vi "update_switch_counter.vi"(0 "PrepLineObject.lvclass":refnum<class "PrepLineObject.lvclass">, 3 "error in (no error)":errorcluster) -> (7 "PrepLineObject out":refnum<class "PrepLineObject.lvclass">, 10 "error out":errorcluster)   [LabVIEW 2018]
doc: "if the switch is turned to true/activated (valve open) the counter in the PrepLineObject is increased by 1. The switch preference file is also being updated"
uses:
  Classes/PrepLineObject/PrepLineObject.lvclass
  <vilib>/Utility/config.llb/Write Key (U32).vi
  <vilib>/Utility/config.llb/NI_LVConfig.lvlib
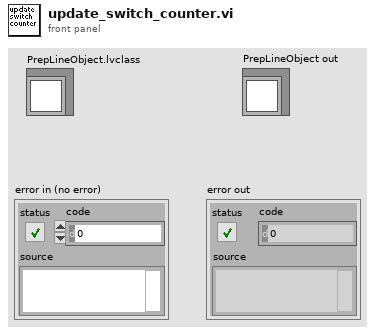
[diagram p1: front panel]
types:
  T1 = typedef "NI_LVConfig.lvlib/Config Data RefNum.ctl" = refnum<k1>
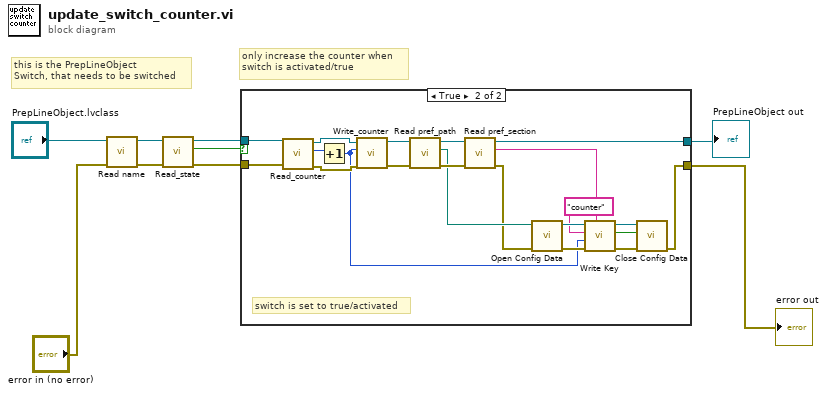
[diagram p0: block diagram]
diagram:
  # "only increase the counter when\nswitch is activated/true"
  # "this is the PrepLineObject\nSwitch, that needs to be switched"
  n1 = call-dynamic "Read name.vi"("error in (no error)"="error in (no error)", "PrepLineObject in"="PrepLineObject.lvclass") -> ("error out"=w7:errorcluster, "PrepLineObject out"=w8:refnum<class "PrepLineObject.lvclass">)  [unwired: 7 in, 1 out]
  n2 = call-dynamic "Read_state.vi"("error in (no error)"=w7, "PrepLineObject in"=w8) -> ("error out"=w5:errorcluster, "state"=w4:bool, "PrepLineObject out"=w6:refnum<class "PrepLineObject.lvclass">)  [unwired: 7 in]
  n3 = case shown="True" w4 {
    tunnel: w6 -> [w11 w29]
    tunnel: w5 -> [w10 w28]
    tunnel: [w11 w23] -> w2
    tunnel: [w10 w12] -> w1
    frame False {
      # "switch is set to false/inactive"
    }
    frame True {
      # "switch is set to true/activated"
      n4 = call-dynamic "Read_counter.vi"("error in (no error)"=w28, "PrepLineObject in"=w29) -> ("error out"=w30:errorcluster, "counter"=w32:u32, "PrepLineObject out"=w31:refnum<class "PrepLineObject.lvclass">)  [unwired: 7 in]
      n5 = Increment(x=w32) -> (x+1=w16:u32)
      n6 = call-dynamic "Write_counter.vi"("error in (no error)"=w30, "counter"=w16, "PrepLineObject in"=w31) -> ("error out"=w26:errorcluster, "PrepLineObject out"=w27:refnum<class "PrepLineObject.lvclass">)  [unwired: 7 in]
      n7 = call-dynamic "Read pref_path.vi"("error in (no error)"=w26, "PrepLineObject in"=w27) -> ("error out"=w24:errorcluster, "pref path"=w22:path, "PrepLineObject out"=w25:refnum<class "PrepLineObject.lvclass">)  [unwired: 7 in]
      n8 = call-dynamic "Read pref_section.vi"("error in (no error)"=w24, "PrepLineObject in"=w25) -> ("error out"=w21:errorcluster, "pref section"=w18:string, "PrepLineObject out"=w23:refnum<class "PrepLineObject.lvclass">)  [unwired: 7 in]
      n9 = call <vilib>:"Open Config Data.vi"("error in (no error)"=w21, "configuration file path"=w22) -> ("error out"=w20:errorcluster, "refnum"=w19:T1)  [unwired: 7 in, 1 out]
      n10 = call-poly <vilib>:"Write Key.vi"("section"=w18, "error in (no error)"=w20, "value"=w16, "key"="counter", "refnum"=w19) -> ("error out"=w15:errorcluster, "found?"=w14:bool, "refnum out"=w13:T1)  [unwired: 4 in]
      n11 = call <vilib>:"Close Config Data.vi"("error in (no error)"=w15, "write file if changed (T)"=w14, "refnum"=w13) -> ("error out"=w12:errorcluster)  [unwired: 7 in, 1 out]
    }
  }
  "error out" <- w1
  "PrepLineObject out" <- w2
